vi "Main Process Outgoing Messages.vi"(8 "error in":errorcluster, 10 "Outgoing Cyclic Configuraiton":T1 {"Outgoing Cyclic Frame"."Transmit Propreties"."Transmit Time" format="%#_p"}, 11 "internal data":T6={"J1939 XNET Settings"={"XNET Database"="", "XNET Cluster"="", "CAN port"="", "Baud rate [Bd]"=0, "J1939 Network Address"=0, "Name"=0, "Termination"=0}, "j1939 queues"={"Processed Outgoing"=refnum, "Process Outgoing"=refnum, "stop notifier"=refnum, "error queue"=refnum, "active dtc"=refnum, "processed inc"=refnum}, "fgv references"={"BAM Buffer"=refnum, "CM Buffer"=refnum, "CM Gen"=refnum, "BAM Gen"=refnum, "Address Claims"=refnum, "RQST"=refnum, "scaling lut"=refnum, "data lut"=refnum, "cyclic scheduler"=refnum}, "frame in"="", "frame out"="", "timing"={"tb to j1939 queue timeout"=100, "j1939 to tb queue timeout"=100, "dtc loop period (ms)"=100, "CAN in loop period (ms)"=100, "process incoming queue timeout (ms)"=100, "Outgoing Write Decimation"=0, "process outgoing loop rate (ms)"=0, "periodic outgoing queue timeout (ms)"=10, "CAN out queue timeout (ms)"=100}}) -> ()   [LabVIEW 2013, in "J1939.lvlib"]
uses:
  J1939.lvlib
  API Types/Internal Data.ctl
  API Types/XNET Settings.ctl
  API Types/Setup Information Cluster.ctl
  API Types/CAN Outgoing Message Cluster.ctl
  API Types/Convert DTCs Cluster.ctl
  <vilib>/xnet/xnet.llb/XNET Frame CAN.ctl
  <vilib>/xnet/xnet.llb/XNET Frame Type CAN.ctl
  TP/TP List References.ctl
  BAM/BAM Buffer Connections List_Ref.ctl
  Connection Mode/Connection Mode Generation Connection Ref.ctl
  BAM/BAM Generation Connections List_Ref.ctl
  LUTs/J1939 Address Table Reference.ctl
  RQST/RQST Lookup Table Reference.ctl
  LUTs/J1939 Conversion Lookup Table Reference.ctl
  LUTs/J1939 Data Lookup Table Reference.ctl
  LUTs/Cyclic Frame Scheduler Lut Reference.ctl
  Configuration/TypeDefs/timing configuration.ctl
  CD/CD Outgoing Cyclic Configuration.ctl
  CD/CD Outgoing Cyclic Frame Pairs.ctl
  API Types/XNET Frame Event Properties.ctl
  module/configuration/Signal Mapping.ctl
  <vilib>/NI/Tag Bus/tag/Data Type.ctl
  API Types/Periodic Message Generator Cluster.ctl
  LUTs/Cyclic Frame Scheduler LUT Command.ctl
  Read Queued Outgoing Messages.vi
  Process Outgoing Messages by Frame Type.vi
  Periodic Message Generator.vi
  Connection Mode/Connection Mode Generation Queue Messages.vi
  Check Output Message Frame Type.vi
  BAM/BAM Generation.vi
  BAM/BAM Generation Connections List_Actions.vi
  BAM/BAM Generation Create New TP Connection.vi
  Connection Mode/Connection Mode Generation.vi
  Connection Mode/Connection Mode Generation Connections List_Actions.vi
  Connection Mode/Connection Mode Generation Search for Connection (Local Message).vi
  Connection Mode/Connection Mode Generation Create New TP Connection.vi
  Convert Signals to Frame by ID.vi
  Connection Mode/Connection Mode Generation Get Next Messages.vi
  Common Messages/J1939 Message TP.Conn Abort.vi
  Frame Conversion/Common Conversions.vi
  Frame Conversion/Convert CAN Arb ID to J1939 ID.vi
  Common Messages/J1939 Common Messages.vi
  Common Messages/J1939 Message TP.CM BAM.vi
  Common Messages/J1939 Message TP.DT.vi
  Common Messages/J1939 Message TP.CM RTS.vi
  Conversion Lookup Table Get Conversion Parameter.vi
  LUTs/J1939 Data Lookup Table Get Signals (Range).vi
  Frame Conversion/Convert J1939 ID to CAN Arb ID.vi
  <vilib>/xnet/xnet.llb/XNET Convert.vi
  <vilib>/xnet/xnet.llb/XNET Convert (Signal to Frame Raw).vi
  BAM/BAM Generation Search for Connection (Local Message).vi
  BAM/BAM Generation Queue Messages.vi
  <vilib>/NI/Tag Bus/tag/tag descriptor.lvclass
  module/configuration/J1939 configuration.lvclass
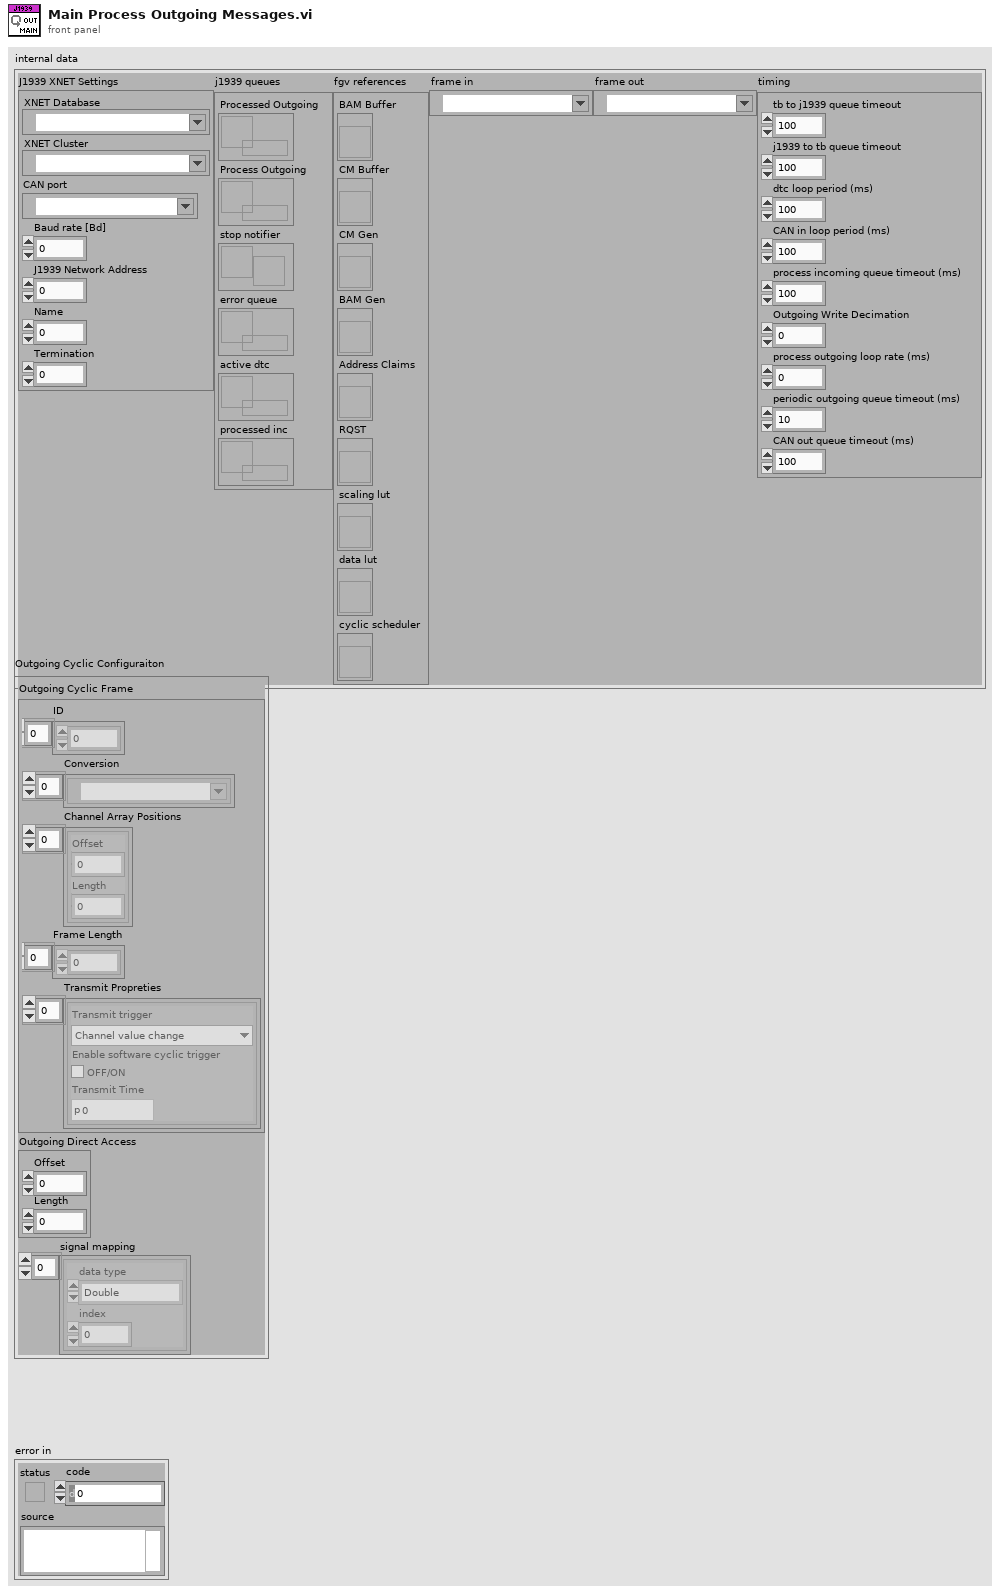
[diagram p1: front panel]
types:
  T1 = typedef "J1939.lvlib/CD Outgoing Cyclic Configuration.ctl" = cluster{"Outgoing Cyclic Frame":T2, "Outgoing Direct Access":cluster{"Offset":u32, "Length":u32}, "signal mapping":T4[]}
  T2 = typedef "J1939.lvlib/CD Outgoing Cyclic Frame Pairs.ctl" = cluster{"ID":u32[], "Conversion":refnum<k21>[], "Channel Array Positions":cluster{"Offset":u32, "Length":u32}[], "Frame Length":u32[], "Transmit Propreties":T3[]}
  T3 = typedef "J1939.lvlib/XNET Frame Event Properties.ctl" = cluster{"Transmit trigger":enum16{"Channel value change"}, "Enable software cyclic trigger":bool, "Transmit Time":dbl}
  T4 = typedef "J1939 configuration.lvclass/Signal Mapping.ctl" = cluster{"data type":T5, "index":i32}
  T5 = typedef "tag bus.lvlib/tag descriptor.lvclass/Data Type.ctl" = enum16{"Double", "Single", "I64", "I32", "I16", "I8", "U64", "U32", "U16", "U8", "Boolean", "String", "Array of Double", "Array of Single", "Array of I64", "Array of I32", "Array of I16", "Array of I8", "Array of U64", "Array of U32", "Array of U16", "Array of U8", "Array of Boolean", "Array of String"}
  T6 = typedef "J1939.lvlib/Internal Data.ctl" = cluster{"J1939 XNET Settings":T7, "j1939 queues":T8, "fgv references":T9, "frame in":refnum<k21>, "frame out":refnum<k21>, "timing":T18}
  T7 = typedef "J1939.lvlib/XNET settings.ctl" = cluster{"XNET Database":refnum<k21>, "XNET Cluster":refnum<k21>, "CAN port":refnum<k21>, "Baud rate [Bd]":u32, "J1939 Network Address":u8, "Name":u64, "Termination":u32}
  T8 = typedef "J1939.lvlib/Setup Information Cluster.ctl" = cluster{"Processed Outgoing":refnum<queue>, "Process Outgoing":refnum<queue>, "stop notifier":refnum<notifier>, "error queue":refnum<queue>, "active dtc":refnum<queue>, "processed inc":refnum<queue>}
  T9 = typedef "J1939.lvlib/TP List References.ctl" = cluster{"BAM Buffer":T10, "CM Buffer":T10, "CM Gen":T11, "BAM Gen":T12, "Address Claims":T13, "RQST":T14, "scaling lut":T15, "data lut":T16, "cyclic scheduler":T17}
  T10 = typedef "J1939.lvlib/BAM Buffer Connections List_Ref.ctl" = refnum<vi>
  T11 = typedef "J1939.lvlib/Connection Mode Generation Connection Ref.ctl" = refnum<vi>
  T12 = typedef "J1939.lvlib/BAM Generation Connections List_Ref.ctl" = refnum<vi>
  T13 = typedef "J1939.lvlib/J1939 Address Table Reference.ctl" = refnum<vi>
  T14 = typedef "J1939.lvlib/RQST Lookup Table Reference.ctl" = refnum<vi>
  T15 = typedef "J1939.lvlib/J1939 Conversion Lookup Table Reference.ctl" = refnum<vi>
  T16 = typedef "J1939.lvlib/J1939 Data Lookup Table Reference.ctl" = refnum<vi>
  T17 = typedef "J1939.lvlib/cyclic frame scheduler lut reference.ctl" = refnum<vi>
  T18 = typedef "J1939.lvlib/timing configuration.ctl" = cluster{"tb to j1939 queue timeout":i32, "j1939 to tb queue timeout":i32, "dtc loop period (ms)":i32, "CAN in loop period (ms)":i32, "process incoming queue timeout (ms)":i32, "Outgoing Write Decimation":u32, "process outgoing loop rate (ms)":i32, "periodic outgoing queue timeout (ms)":i32, "CAN out queue timeout (ms)":i32}
  T19 = typedef "J1939.lvlib/cyclic frame scheduler lut command.ctl" = enum16{"Initialize", "set", "remove", "calculate times"}
  T20 = typedef "J1939.lvlib/Periodic Message Generator Cluster.ctl" = cluster{"Arb ID":u32, "Timeout":u32, "Start Timeout":u32}
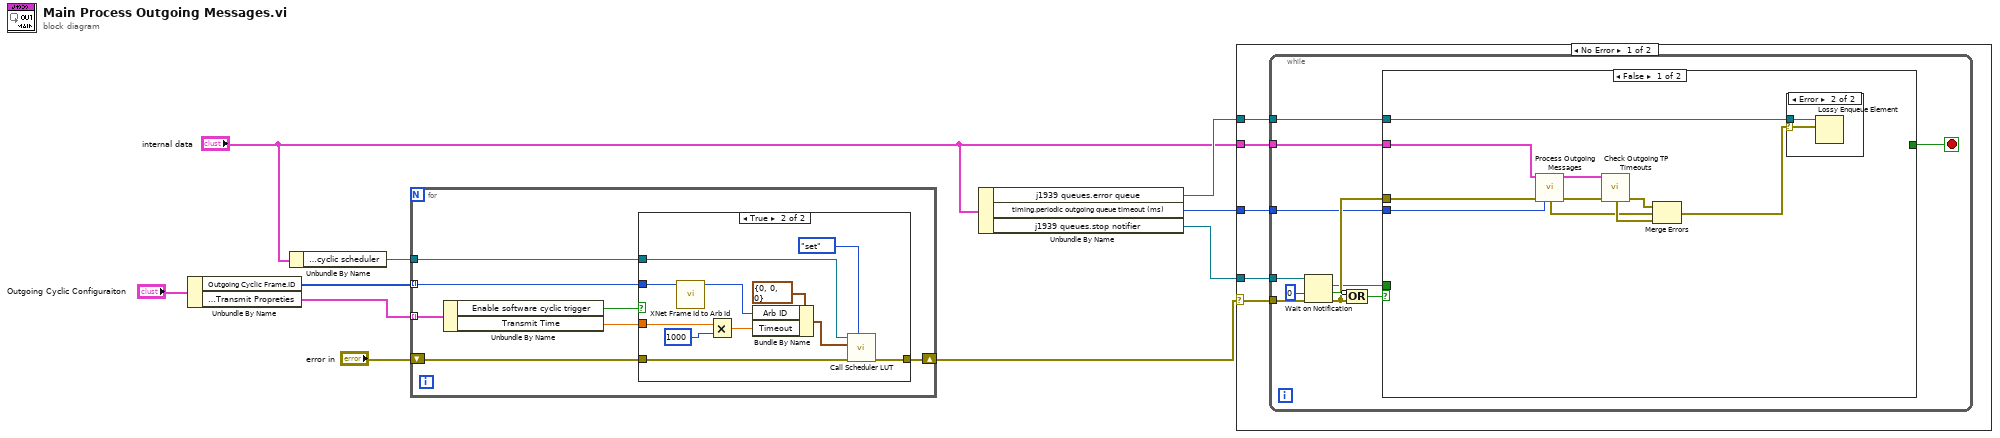
[diagram p0: block diagram]
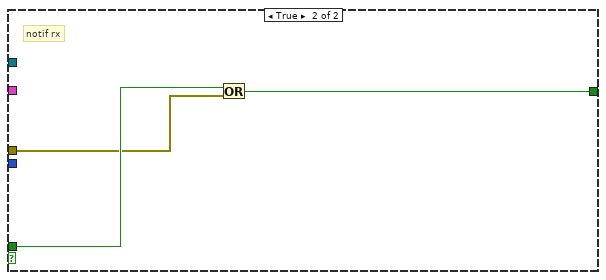
[diagram p3: hidden frame]
diagram:
  n1 = Unbundle By Name("Outgoing Cyclic Configuraiton") -> ("Outgoing Cyclic Frame.ID"=w9:u32[], "Outgoing Cyclic Frame.Transmit Propreties"=w8:T3[])
  n2 = Unbundle By Name("internal data") -> ("fgv references.cyclic scheduler"=w3:T17)
  n3 = for {
    tunnel: w9 -> [w17] mode=indexing
    tunnel: w8 -> [w16] mode=indexing
    tunnel: w3 -> [w11]
    shift-right: [w12] -> w1
    shift-left: "error in" -> [w13]
    n4 = Unbundle By Name(w16) -> ("Enable software cyclic trigger"=w15:bool, "Transmit Time"=w14:dbl)
    n5 = case shown="True" w15 {
      tunnel: w17 -> [_ w20]
      tunnel: w14 -> [_ w27]
      tunnel: w13 -> [w18 w24]
      tunnel: [w18 w25] -> w12
      tunnel: w11 -> [_ w23]
      frame False {
      }
      frame True {
        n6 = call "XNet Frame Id to Arb Id.vi"("ID"=w20) -> ("Arb id"=w19:u32)  [unwired: 10 in]
        n7 = Multiply(x=w27, y=1000) -> (x*y=w26:dbl)
        n8 = Bundle By Name(cluster=T20 {"Arb ID"=0, "Timeout"=0, "Start Timeout"=0}, "Arb ID"=w19, "Timeout"=w26) -> (w22:T20)
        n9 = call "Call Scheduler LUT.vi"("command"=cyclic_frame_scheduler_lut_command."set", "error in"=w24, "frame schedule"=w22, "scheduler lut"=w23) -> ("error out"=w25:errorcluster)  [unwired: 6 in, 1 out]
      }
    }
  }
  n10 = Unbundle By Name("internal data") -> ("j1939 queues.error queue"=w6:refnum<queue>, "timing.periodic outgoing queue timeout (ms)"=w5:i32, "j1939 queues.stop notifier"=w7:refnum<notifier>)
  n11 = case shown="No Error" w1 {
    selector: w1 -> [w34 _]
    tunnel: w7 -> [w33 _]
    tunnel: "internal data" -> [w32 _]
    tunnel: w6 -> [w31 _]
    tunnel: w5 -> [w30 _]
    frame No Error {
      n12 = while {
        tunnel: w33 -> [w44]
        tunnel: w34 -> [w45]
        tunnel: w32 -> [w37]
        tunnel: w31 -> [w36]
        tunnel: w30 -> [w35]
        stop <- w39 stop-if-true
        n13 = Wait on Notification(notifier=w44, timeout in ms (-1)=0, error in (no error)=w45) -> (notification=w40:bool, timed out?=w43:bool, error out=w41:errorcluster)  [unwired: 1 in, 1 out]
        n14 = Compound Arithmetic op=OR(invert w43, w41) -> (w42:bool)
        n15 = case shown="False" w42 {
          tunnel: w41 -> [w51 w58]
          tunnel: w40 -> [_ w60]
          tunnel: [_ w59] -> w39
          tunnel: w37 -> [w50 _]
          tunnel: w36 -> [w49 _]
          tunnel: w35 -> [w46 _]
          frame False {
            n16 = call "Process Outgoing Messages.vi"("internal data"=w50, "error in"=w51, "timeout in ms (-1)"=w46) -> ("internal data out"=w47:T6, "Message Errors"=w53:errorcluster, "error out"=w52:errorcluster)  [unwired: 1 in, 9 out]
            n17 = call "Check Outgoing TP Timeouts.vi"("internal data"=w47, "error in"=w52) -> ("Message Error"=w54:errorcluster, "error out"=w55:errorcluster)  [unwired: 1 in, 11 out]
            n18 = Merge Errors(w55, w53, w54) -> (w48:errorcluster)
            n19 = case shown="Error" w48 {
              selector: w48 -> [_ w56]
              tunnel: w49 -> [_ w57]
              frame No Error {
              }
              frame Error {
                n20 = Lossy Enqueue Element(queue=w57, element=w56) -> ()  [unwired: 1 in, 4 out]
              }
            }
          }
          frame True {
            # "notif rx"
            n21 = Or(x=w60, y=w58) -> (x .or. y?=w59:bool)
          }
        }
      }
    }
    frame Error {
    }
  }
